vi "String.Spreadsheet String to 1D Array.vi"(8 "error in":errorcluster, 11 "CSV String":string) -> (0 "error out":errorcluster, 3 "Array":string[](array[string]))   [LabVIEW 2018]
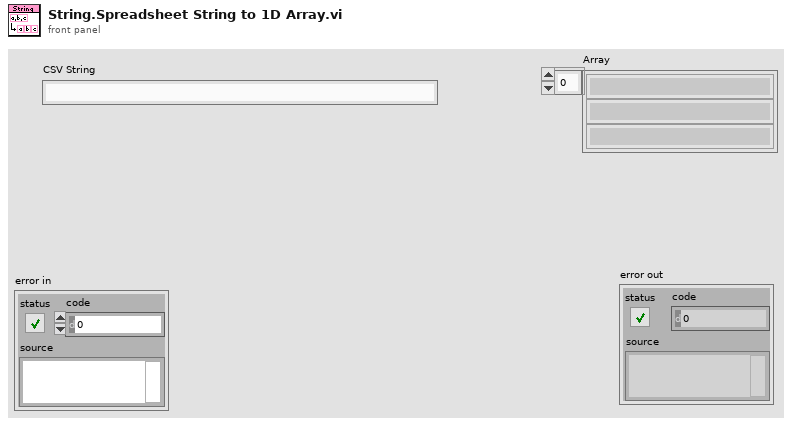
[diagram p1: front panel]
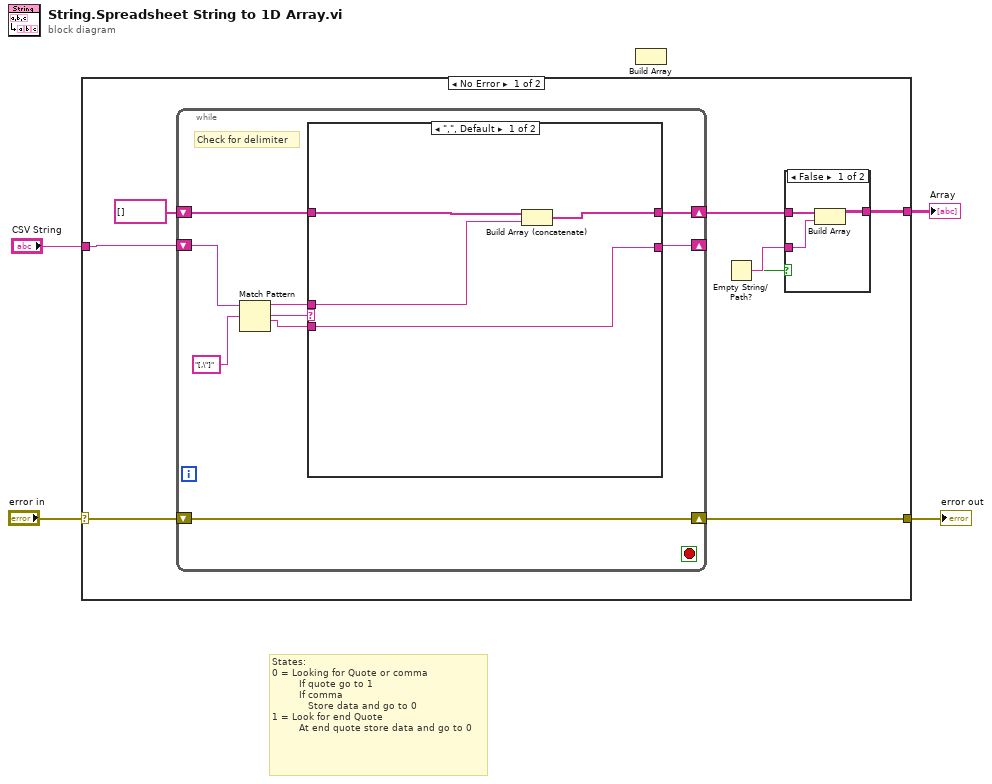
[diagram p0: block diagram]
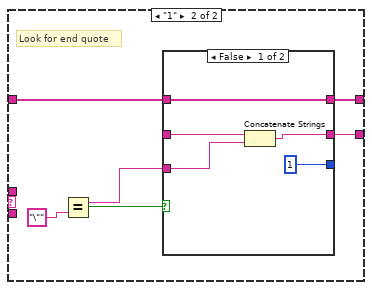
[diagram p2: hidden frame]
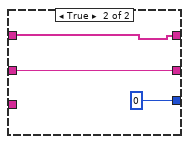
[diagram p3: hidden frame]
diagram:
  # "States:\n0 = Looking for Quote or comma\n         If quote go to 1\n         If comma\n            Store data and go to 0\n1 = Look for end Quote\n         At end quote store data and go to 0"
  n1 = case shown="No Error" "error in" {
    selector: "error in" -> [w12 w44]
    tunnel: [w11 w44] -> w3
    tunnel: "CSV String" -> [w5 _]
    tunnel: [w9 _] -> w1
    frame No Error {
      n2 = while {
        shift-right: [w21] -> w11
        shift-left: w12 -> [w21]
        shift-right: [w19] -> w8
        shift-left: string[] [] -> [w20]
        shift-right: [w13] -> _
        shift-left: w5 -> [w18]
        stop <- _ stop-if-true
        # "Check for delimiter"
        n3 = Match Pattern(string=w18, regular expression="[,\"]") -> (before substring=w15:string, match substring=w16:string, after substring=w14:string)  [unwired: 1 in, 1 out]
        n4 = case shown="\",\", Default" w16 {
          tunnel: [w22 w29] -> w13
          tunnel: w20 -> [w25 w28]
          tunnel: [w24 w27] -> w19
          tunnel: w15 -> [w23 _]
          tunnel: w14 -> [w22 _]
          frame ",", Default {
            n5 = Build Array (concatenate)(w25, w23) -> (w24:string[])
          }
          frame "1" {
            # "Look for end quote"
            n6 = Equal?(y="\"") -> (x=w26:string, x = y?=w30:bool)
            n7 = case shown="False" w30 {
              tunnel: [1 0] -> _
              tunnel: _ -> [w36 w37]
              tunnel: [w35 w37] -> w29
              tunnel: w28 -> [w33 w38]
              tunnel: [w33 w38] -> w27
              tunnel: w26 -> [w34 _]
              frame False {
                n8 = Concatenate Strings(w36, w34) -> (w35:string)
              }
              frame True {
              }
            }
          }
        }
      }
      n9 = Empty String/Path?() -> (string/path=w7:string, empty?=w6:bool)
      n10 = case shown="False" w6 {
        tunnel: [w42 w43] -> w9
        tunnel: w8 -> [w41 w43]
        tunnel: w7 -> [w40 _]
        frame False {
          n11 = Build Array(w41, w40) -> (w42:string[][])
        }
        frame True {
        }
      }
    }
    frame Error {
    }
  }
  "Array" <- w1
  "error out" <- w3
  n12 = Build Array() -> ()  [unwired: 2 in, 1 out]
